vi "2 - DAQmx Bus Analog Input.vi"() -> ()   [LabVIEW 2021]
uses:
  <vilib>/TSA/Omni-Bus/Omni-Bus/Omni_Bus.lvclass
  <vilib>/TSA/Omni-Bus/Omni-Bus/Support/Broad Types.ctl
  <vilib>/TSA/Abstract Data Classes/Abs_Types/Type/Abs_Type.lvclass/Abs_Type.ctl
  <vilib>/TSA/Omni-Bus/Omni-Bus/Omni_Bus.lvclass/Omni_Bus.ctl
  <vilib>/TSA/Omni-Bus/Omni-Bus/Support/Read/Read DBL.vi
  <vilib>/TSA/Omni-Bus/Omni-Bus/Support/FindVar.vi
  <vilib>/Utility/error.llb/Clear Errors.vi
  <vilib>/TSA/Omni-Bus/Omni-Bus/Properties/Read Var Map.vi
  <vilib>/TSA/Abstract Data Classes/Abs_Types/Type/Properties/Read Tag.vi
  DAQmx-Bus.lvclass
  C:/Program Files (x86)/National Instruments/LabVIEW 2021/vi.lib/TSA/Omni-Bus/Omni-Bus/Bus Access/Bus_Access.lvclass
  <vilib>/TSA/Abstract Data Classes/Abs_Types/Double Float/Abs_Double Float.lvclass
  C:/Program Files (x86)/National Instruments/LabVIEW 2021/vi.lib/TSA/Abstract Data Classes/Abs_Types/Type/Abs_Type.lvclass
  <vilib>/TSA/Abstract Data Classes/Abs_Types/Value/Abs_Value.lvclass
  <vilib>/TSA/Omni-Bus/Omni-Bus/Support/Check For Read Only Error.vi
  <vilib>/TSA/Omni-Bus/Omni-Bus/Support/Incorrect Tag String Error.vi
  <vilib>/TSA/Abstract Data Classes/Abs_Types/Type/Abs_Type.lvclass
panel:
  in  "DAQmx Task":refnum<k21>="MyVoltageTask"
  out "timed out?":bool
  in  "stop":bool
  out "Gauge":dbl(knob) scale=-10.0..10.0
  in  "Analog Input Tag":string(combo)
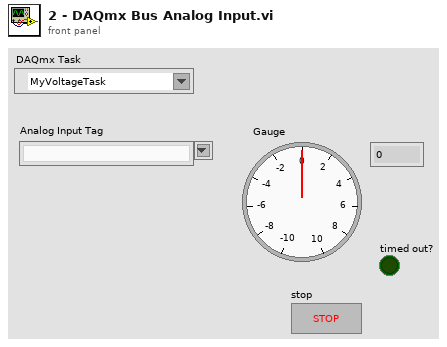
[diagram p1: front panel]
types:
  T1 = typedef "Omni_Bus.lvclass/Broad Types.ctl" = enum16{"All Tags", "NI Specific Type", "Boolean", "String", "Numeric", "Float", "Integer", "Collection", "All Value Types", "Non Value Types"}
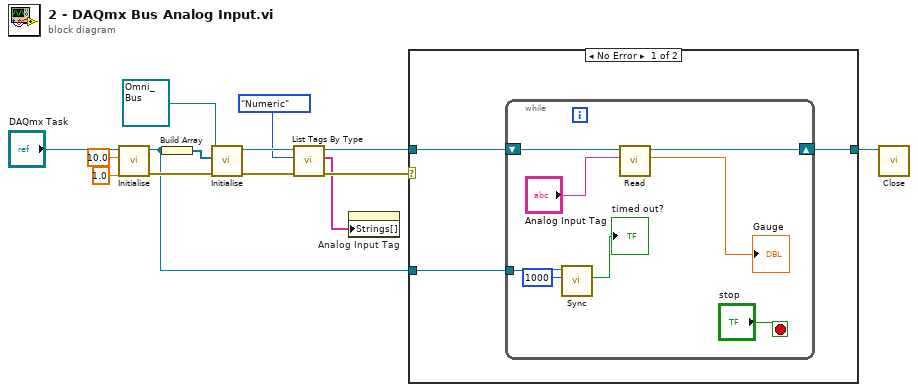
[diagram p0: block diagram]
diagram:
  n1 = call "Initialise.vi"("Update Rate (Hz) - Non HW Timed"=1.0, "timeout (s)"=10.0 ("timeout"), "DAQmx Task"="DAQmx Task") -> ("error out"=w10:errorcluster, "DAQmx-Bus out"=w2:refnum<class "DAQmx-Bus.lvclass">)  [unwired: 7 in]
  n2 = Build Array(w2) -> (w12:refnum<class "DAQmx-Bus.lvclass">[])
  n3 = call-dynamic "Initialise.vi"("error in (no error)"=w10, "Bus Access"=w12, "Var Bus in"=refnum<class "Omni_Bus.lvclass"> refnum) -> ("error out"=w7:errorcluster, "Var Bus out"=w8:refnum<class "Omni_Bus.lvclass">)  [unwired: 7 in]
  n4 = call <vilib>:"List Tags By Type.vi"("error in (no error)"=w7, "Broad Types"=Broad_Types."Numeric", "Var Bus in"=w8) -> ("error out"=w5:errorcluster, "Tags"=w4:string[], "Var Bus out"=w6:refnum<class "Omni_Bus.lvclass">)  [unwired: 5 in, 1 out]
  n5 = property on="Analog Input Tag" class="CmbBox"("Strings[]"=w4) -> ()  [unwired: 2 in, 2 out]
  n6 = case shown="No Error" w5 {
    tunnel: [w17 w26] -> w9
    tunnel: w6 -> [w16 w26]
    tunnel: w2 -> [w15 _]
    frame No Error {
      n7 = while {
        shift-right: [w25] -> w17
        shift-left: w16 -> [w24]
        tunnel: w15 -> [w20]
        stop <- "stop" stop-if-true
        n8 = call-dynamic "Sync.vi"("timeout in ms (-1)"=1000, "DAQmx-Bus in"=w20) -> ("timed out?"=→"timed out?":bool)  [unwired: 7 in, 2 out]
        n9 = call-poly <vilib>:"Read.vi"("Tag"="Analog Input Tag", "Var Bus in"=w24) -> ("Numeric"=→"Gauge":dbl, "Var Bus out"=w25:refnum<class "Omni_Bus.lvclass">)  [unwired: 7 in, 1 out]
      }
    }
    frame Error {
    }
  }
  n10 = call-dynamic "Close.vi"("Data in"=w9) -> ()  [unwired: 9 in, 2 out]
